vi "Global 2.vi"() -> ()   [LabVIEW 2022 SP3]
panel:
  in  "OK Button":bool
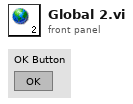
[diagram p1: front panel]
diagram:
